vi "NewLayoutFromExistingDialog.vi"(10 "Layout Ring Refnum":refnum<vi>) -> (1 "Based on":i32(ring), 2 "New Layout name":string, 3 "Cancelled?":bool)   [LabVIEW 2013]
uses:
  <vilib>/Utility/miscctls.llb/LVStringsAndValuesArrayTypeDef_I32.ctl
panel:
  in  "Cancel Button":bool
  in  "OK Button":bool
  in  "Based on existing:":i32(ring) items=["(present)"=-2, ""=0]
  in  "New Layout name:":string
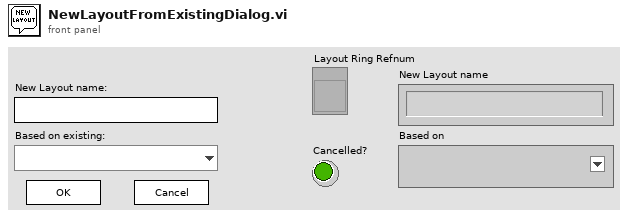
[diagram p1: front panel]
types:
  T1 = enum8{"Enabled", "Disabled", "Disabled and Grayed Out"}
  T2 = typedef "LVStringsAndValuesArrayTypeDef_I32.ctl" = cluster{"String":string, "Value":i32}[]
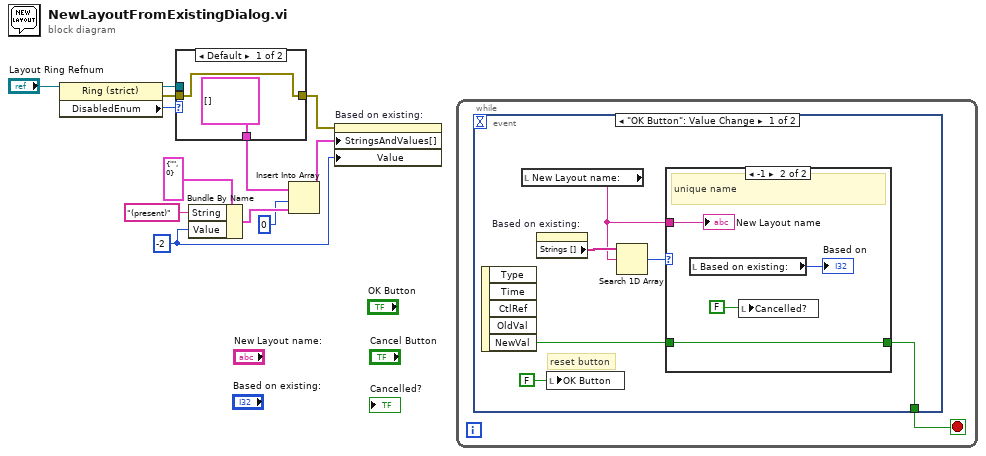
[diagram p0: block diagram]
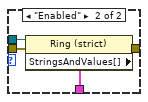
[diagram p2: hidden frame]
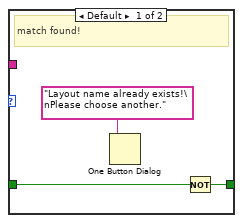
[diagram p3: hidden frame]
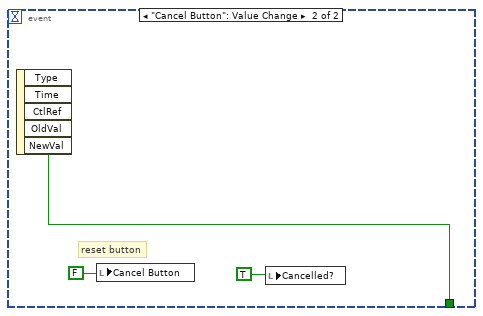
[diagram p4: hidden frame]
diagram:
  w7 = -2 ("Value")
  n1 = property class="Ring (strict)"(reference="Layout Ring Refnum") -> (reference out=w3:refnum<vi>, error out=w2:errorcluster, "DisabledEnum"=w1:T1)  [unwired: 1 in]
  n2 = case shown="Default" w1 {
    tunnel: [w14 w18] -> w12
    tunnel: [T2 [] ("StringsAndValues[]") w17] -> w11
    tunnel: w3 -> [_ w16]
    tunnel: w2 -> [w14 w15]
    frame Default {
    }
    frame "Enabled" {
      n3 = property class="Ring (strict)"(reference=w16, error in=w15) -> (error out=w18:errorcluster, "StringsAndValues[]"=w17:T2)  [unwired: 1 out]
    }
  }
  n4 = Bundle By Name(cluster=cluster{"String":string, "Value":i32} {"String"="", "Value"=0}, "String"="(present)", "Value"=w7) -> (w9:cluster{"String":string, "Value":i32})
  n5 = Insert Into Array(array=w11, index=0, new element=w9) -> (w6:T2)
  n6 = property on="Based on existing:" class="Ring (strict)"(error in=w12, "StringsAndValues[]"=w6, "Value"=w7) -> ()  [unwired: 1 in, 2 out]
  n7 = while {
    stop <- w19 stop-if-true
    n8 = event shown="[0] \"OK Button\": Value Change" {
      selector: _ -> [_ _]
      dyn-events: _ -> [_ _]
      timeout: _ -> [_ _]
      tunnel: [w22 w34] -> w19
      event "OK Button": Value Change {
        # "reset button"
        n9 = event-data() -> ("NewVal"=w21:bool)  [unwired: 1 in, 4 out]
        n10 = local read "New Layout name:"() -> (w24:string)
        n11 = property on="Based on existing:" class="Ring (strict)"() -> ("Strings []"=w25:string[])  [unwired: 2 in, 2 out]
        n12 = local write "OK Button"(FALSE) -> ()
        n13 = Search 1D Array(1D array=w25, element=w24) -> (index of element=w23:i32)  [unwired: 1 in]
        n14 = case shown="-1" w23 {
          tunnel: w24 -> [_ w30]
          tunnel: w21 -> [w26 w29]
          tunnel: [w28 w29] -> w22
          frame Default {
            # "match found!"
            n15 = One Button Dialog(message="Layout name already exists!\nPlease choose another.") -> ()  [unwired: 1 in, 1 out]
            n16 = Not(x=w26) -> (.not. x?=w28:bool)
          }
          frame -1 {
            # "unique name"
            n17 = local read "Based on existing:"() -> (→"Based on":i32)
            n18 = local write "Cancelled?"(FALSE) -> ()
            "New Layout name" <- w30
          }
        }
      }
      event "Cancel Button": Value Change {
        # "reset button"
        n19 = event-data() -> ("NewVal"=w34:bool)  [unwired: 1 in, 4 out]
        n20 = local write "Cancel Button"(FALSE) -> ()
        n21 = local write "Cancelled?"(TRUE) -> ()
      }
    }
  }
